vi "phone database.vi"() -> ()   [LabVIEW 2011]
uses:
  <vilib>/addons/database/Auxilliary.llb/DB Tools DataTypes.ctl
  <vilib>/addons/database/Auxilliary.llb/DB Tools Cursor Type.ctl
  <vilib>/addons/database/Connection.llb/DB Tools Open Connec (Path).vi
  <vilib>/addons/database/Connection.llb/Conn Execute.vi
  <vilib>/addons/database/Recordset.llb/Rec Fetch Recordset Data (R).vi
  <vilib>/addons/database/Recordset.llb/Rec Destroy - Connection.vi
  <vilib>/addons/database/_DB Variant To Data/Database Variant To Data.xnode
  <vilib>/addons/database/NI_Database_API.lvlib
panel:
  out "data 3":cluster{i32, string, string, string, string}[](array[cluster])
  out "tables":string[](array[string])
  out "data 2":cluster{i32, string, string, string, string}[](array[cluster])
  out "data":variant[][](array[variant])
  out "column information":T2(array[cluster])
  out "columns":string[](array[string])
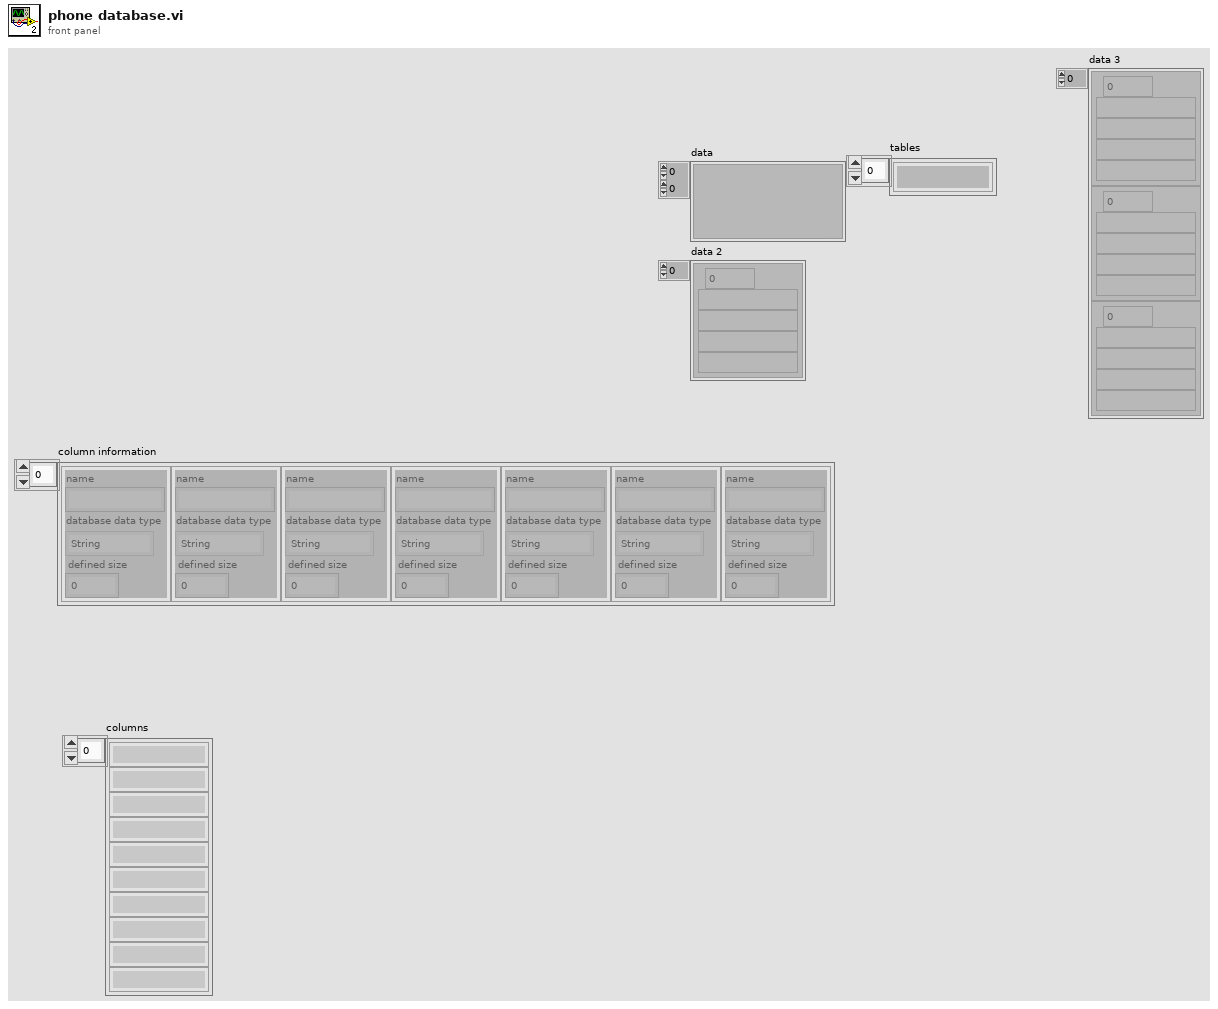
[diagram p1: front panel]
types:
  T1 = typedef "NI_Database_API.lvlib/DB Tools DataTypes.ctl" = enum16{"String", "Long (I32)", "Single (SGL)", "Double (DBL)", "Date/Time", "Binary"}
  T2 = cluster{"name":string, "database data type":T1, "defined size":i32}[]
  T3 = cluster{"id":i32, "num":string, "code":string, "city":string, "cardtype":string}
  T4 = typedef "NI_Database_API.lvlib/DB Tools Cursor Type.ctl" = enum16{"forward-only", "keyset", "dynamic", "static"}
  T5 = typedef "NI_Database_API.lvlib/Conn ObjectReference.ctl" = refnum<k1>
  T6 = cluster{"id":i32, "num":string, "code":string, "city":string, "cardtype":string}[]
  T7 = typedef "NI_Database_API.lvlib/Rec ObjectReference.ctl" = refnum<k1>
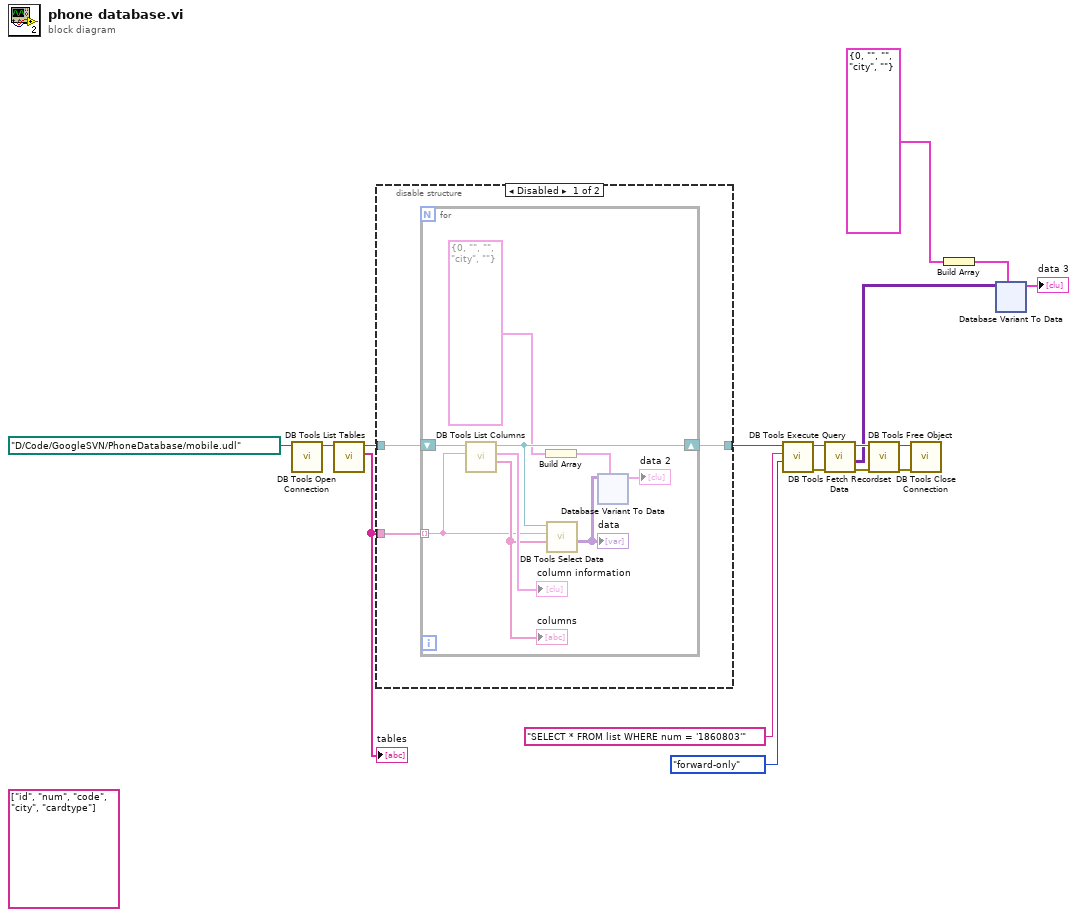
[diagram p0: block diagram]
diagram:
  (unwired) string[] ["id", "num", "code", "city", "cardtype"] ("columns 2")
  n1 = call-poly <vilib>:"DB Tools Open Connection.vi"("connection information"=path "D:/Code/GoogleSVN/PhoneDatabase/mobile.udl") -> ("connection reference"=w14:T5)  [unwired: 7 in, 1 out]
  n2 = call <vilib>:"DB Tools List Tables.vi"("connection reference"=w14) -> ("tables"=w16:string[], "connection reference out"=w15:T5)  [unwired: 4 in, 1 out]
  "tables" <- w16
  n3 = disable-structure shown="Disabled" {
    disable-tunnel: w16 -> [w20 _]
    disable-tunnel: w15 -> [w19 w195]
    disable-tunnel: [w18 w195] -> w13
    frame Disabled {
      n4 = for {
        tunnel: w20 -> [w25] mode=indexing
        shift-right: [w27] -> w18
        shift-left: w19 -> [w29]
        n5 = call <vilib>:"DB Tools List Columns.vi"("table"=w25, "connection reference"=w29) -> ("columns"=w26:string[], "column information"=→"column information":T2, "connection reference out"=w27:T5)  [unwired: 2 in, 1 out]
        "columns" <- w26
        n6 = Build Array(T3 {"id"=0, "num"="", "code"="", "city"="city", "cardtype"=""}) -> (w23:T6)
        n7 = call <vilib>:"DB Tools Select Data.vi"("columns"=w26, "table"=w25, "connection reference"=w27) -> ("data"=w22:variant[][])  [unwired: 3 in, 2 out]
        "data" <- w22
        n8 = xnode "Database Variant To Data"("database variant"=w22, "type"=w23) -> ("data"=→"data 2":cluster{i32, string, string, string, string}[])  [unwired: 1 in, 1 out]
      }
    }
    frame Enabled {
    }
  }
  n9 = call-poly <vilib>:"DB Tools Execute Query.vi"("cursor type"=DB_Tools_Cursor_Type."forward-only", "SQL query"="SELECT * FROM list WHERE num = '1860803'", "connection reference"=w13) -> ("error out"=w9:errorcluster, "recordset reference"=w12:T7)  [unwired: 5 in]
  n10 = call-poly <vilib>:"DB Tools Fetch Recordset Data.vi"("error in (no error)"=w9, "recordset reference"=w12) -> ("error out"=w8:errorcluster, "recordset data"=w1:variant[][], "recordset reference out"=w11:T7)  [unwired: 3 in]
  n11 = call-poly <vilib>:"DB Tools Free Object.vi"("error in (no error)"=w8, "recordset reference"=w11) -> ("error out"=w7:errorcluster, "connection reference"=w10:T5)  [unwired: 8 in]
  n12 = call <vilib>:"DB Tools Close Connection.vi"("error in (no error)"=w7, "connection reference"=w10) -> ()  [unwired: 5 in, 1 out]
  n13 = Build Array(T3 {"id"=0, "num"="", "code"="", "city"="city", "cardtype"=""}) -> (w3:T6)
  n14 = xnode "Database Variant To Data"("database variant"=w1, "type"=w3) -> ("data"=→"data 3":T6)  [unwired: 1 in, 1 out]
